vi "Read Branch Rate - With Two Methods - Returns Total Value.vi"() -> ()   [LabVIEW 2017, in "Cobertura.Tests.lvlib" / "Package.lvlib"]
uses:
  Package.lvlib
  Cobertura/Package/Package.lvclass/Package.ctl
  Cobertura/Package/Read Branch Rate.vi
  <vilib>/PNR/Transparent Assertions/Transparent Assertions/Transparent Assertions.lvlib
  Cobertura/Class/Class.lvclass
  Cobertura/Method/Method.lvclass
  Cobertura/Package/Package.lvclass
panel:
  out "error out":errorcluster
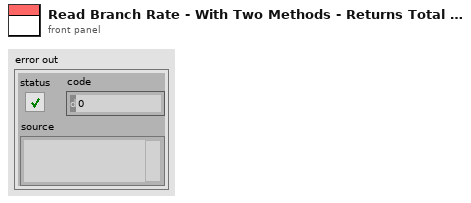
[diagram p1: front panel]
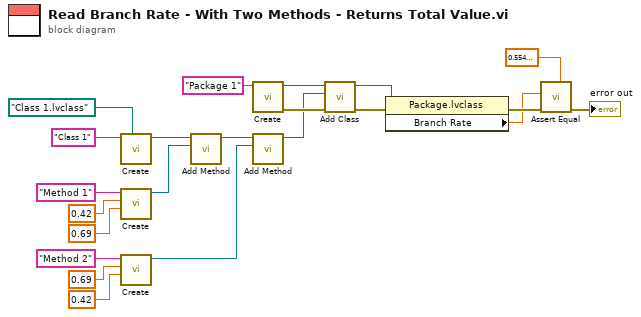
[diagram p0: block diagram]
diagram:
  n1 = call "Create.vi"("Filename"=path "Class 1.lvclass", "Name"="Class 1") -> ("Class"=w18:refnum<class "Class.lvclass">)  [unwired: 8 in, 1 out]
  n2 = call "Create.vi"("Branch Rate"=0.69, "Line Rate"=0.42, "Name"="Method 1") -> ("Method"=w14:refnum<class "Method.lvclass">)  [unwired: 7 in, 1 out]
  n3 = call "Create.vi"("Branch Rate"=0.42, "Line Rate"=0.69, "Name"="Method 2") -> ("Method"=w9:refnum<class "Method.lvclass">)  [unwired: 7 in, 1 out]
  n4 = call "Add Method.vi"("Method"=w14, "Class in"=w18) -> ("Class out"=w10:refnum<class "Class.lvclass">)  [unwired: 8 in, 1 out]
  n5 = call "Create.vi"("Name"="Package 1") -> ("error out"=w4:errorcluster, "Package"=w5:refnum<class "Package.lvclass">)  [unwired: 9 in]
  n6 = call "Add Method.vi"("Method"=w9, "Class in"=w10) -> ("Class out"=w3:refnum<class "Class.lvclass">)  [unwired: 8 in, 1 out]
  n7 = call "Add Class.vi"("error in (no error)"=w4, "Class"=w3, "Package in"=w5) -> ("error out"=w1:errorcluster, "Package out"=w2:refnum<class "Package.lvclass">)  [unwired: 7 in]
  n8 = property class="Package.lvclass"(reference=w2, error in=w1) -> (error out=w21:errorcluster, "Branch Rate"=w8:dbl)  [unwired: 1 out]
  n9 = call <vilib>:"Assert Equal.vi"("Expected"=0.5549999999999999 ("Branch Rate"), "error in (no error)"=w21, "Actual"=w8) -> ("error out"=→"error out":errorcluster)  [unwired: 8 in]
